vi "Serialize Connection Info.vi"(7 "Field Delimiter (::)":string="::", 8 "error in (no error)":errorcluster, 11 "Connection Info":T1={"VISA Resource"="", "Address"=1} {"Address" min=1}) -> (0 "error out 2":errorcluster, 3 "Serialized Connection Info":string)   [LabVIEW 2020, in "plugin_flodx_pressure.lvlib" / "plugin.lvlib" / "Instrument Manager.lvlib"]
doc: "Serializes the connection info. By default, it serializes to the string \"<visa_resource>::<pump_address>\"."
uses:
  Instrument Manager.lvlib
  Connection Info.ctl
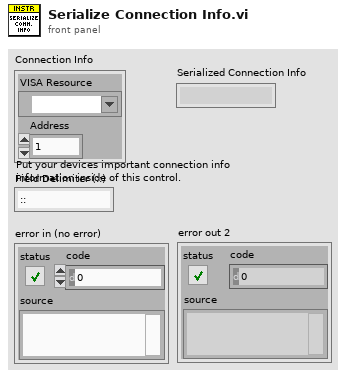
[diagram p1: front panel]
types:
  T1 = typedef "plugin_flodx_pressure.lvlib/plugin.lvlib/Instrument Manager.lvlib/Connection Info.ctl" = cluster{"VISA Resource":refnum<visa-resource-name>, "Address":u8}
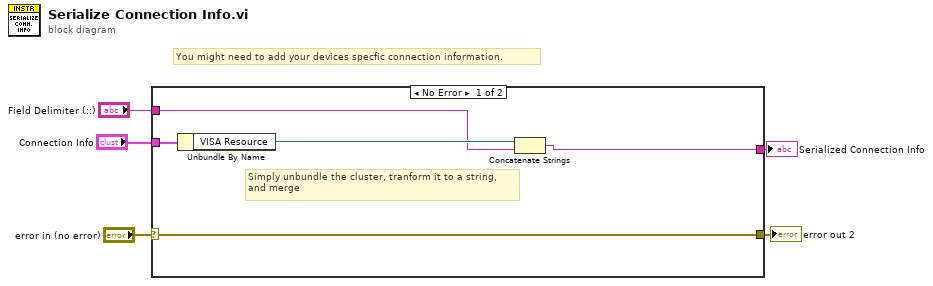
[diagram p0: block diagram]
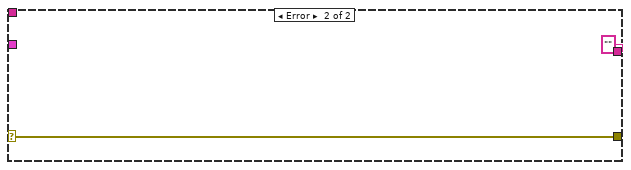
[diagram p2: hidden frame]
diagram:
  # "You might need to add your devices specfic connection information."
  n1 = case shown="No Error" "error in (no error)" {
    selector: "error in (no error)" -> [w10 w12]
    tunnel: [w10 w12] -> w4
    tunnel: "Connection Info" -> [w9 _]
    tunnel: "Field Delimiter (::)" -> [w6 _]
    tunnel: [w8 ""] -> w2
    frame No Error {
      # "Simply unbundle the cluster, tranform it to a string,\nand merge"
      n2 = Unbundle By Name(w9) -> ("VISA Resource"=w7:refnum<visa-resource-name>)
      n3 = Concatenate Strings(w7, w6) -> (w8:string)
    }
    frame Error {
    }
  }
  "error out 2" <- w4
  "Serialized Connection Info" <- w2
